vi "Connection String.vi"(8 "error in (no error)":errorcluster, 11 "SQL Server in":refnum<class "SQL Server.lvclass">) -> (0 "error out":errorcluster, 2 "Connected String":string, 3 "SQL Server out":refnum<class "SQL Server.lvclass">)   [LabVIEW 2021, in "SQL Server.lvclass"]
uses:
  <userlib>/John_Lib/DataBase/SQL Server/SQL Server.lvclass
  <userlib>/John_Lib/DataBase/SQL Server/SQL Server.lvclass/SQL Server.ctl
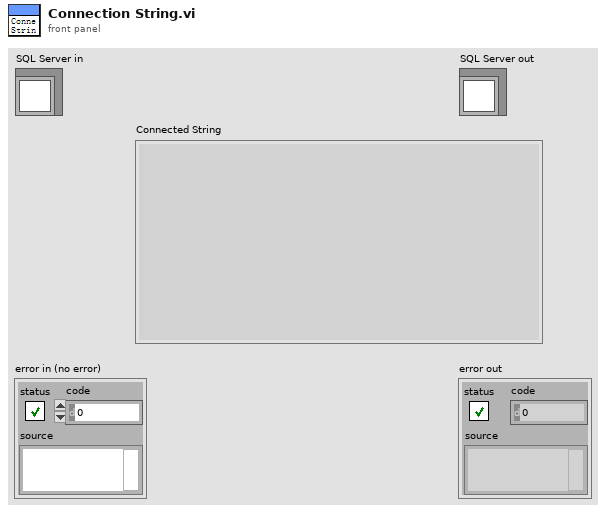
[diagram p1: front panel]
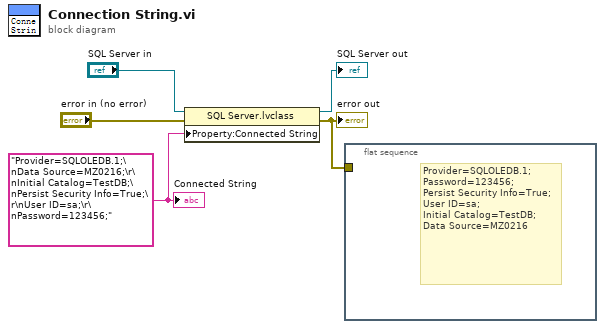
[diagram p0: block diagram]
diagram:
  w3 = "Provider=SQLOLEDB.1;\nData Source=MZ0216;\r\nInitial Catalog=TestDB;\nPersist Security Info=True;\r\nUser ID=sa;\r\nPassword=123456;" ("String")
  n1 = property class="SQL Server.lvclass"(reference="SQL Server in", error in="error in (no error)", "Property:Connected String"=w3) -> (reference out=→"SQL Server out":refnum<class "SQL Server.lvclass">, error out=w1:errorcluster)
  "error out" <- w1
  n2 = flat-sequence {
    tunnel: w1 -> [_]
    frame #0 {
      # "Provider=SQLOLEDB.1;\nPassword=123456;\nPersist Security Info=True;\nUser ID=sa;\nInitial Catalog=TestDB;\nData Source=MZ0216"
    }
  }
  "Connected String" <- w3
